vi "Tank.vi"() -> ()   [LabVIEW 2018]
panel:
  out "Remplissage":u16
  in  "Débit":u16(slide) scale=0.0..10.0
  in  "Consigne":u16(slide) max=1 step=1 scale=1.0..1000.0
  out "Tank":u16(slide) scale=0.0..1000.0
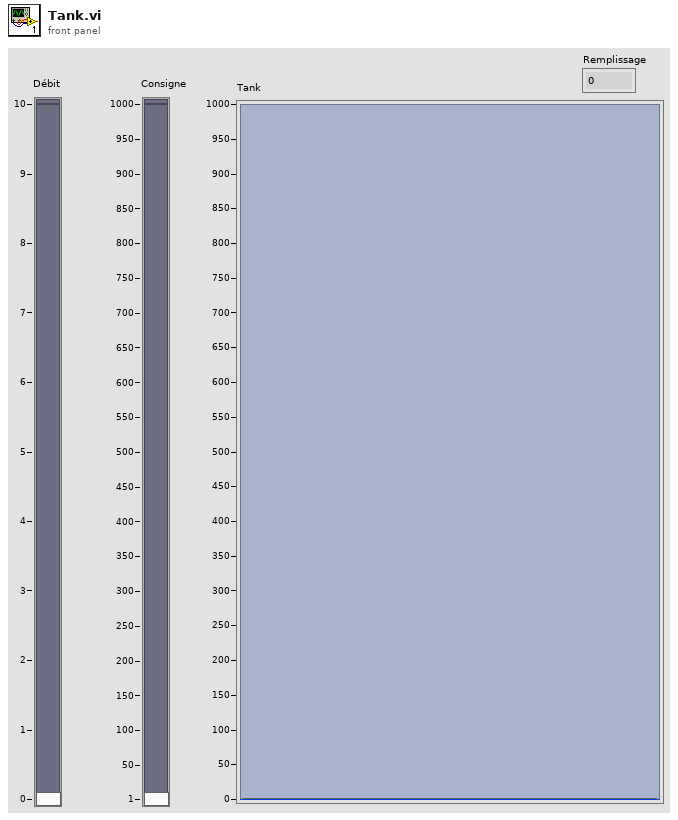
[diagram p1: front panel]
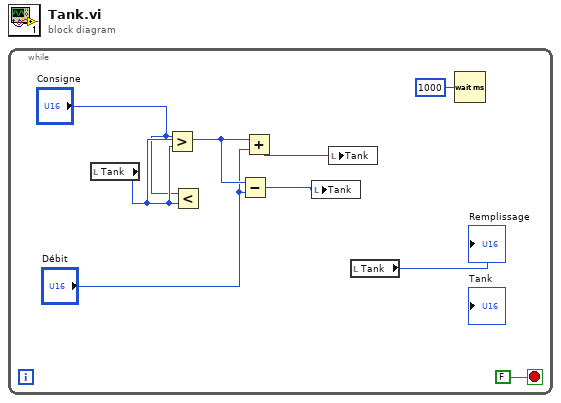
[diagram p0: block diagram]
diagram:
  n1 = while {
    stop <- FALSE stop-if-true
    n2 = local read "Tank"() -> (w6:u16)
    n3 = Greater?(x="Consigne", y=w6) -> ()  [unwired: 1 out]
    n4 = Less?(x="Consigne", y=w6) -> ()  [unwired: 1 out]
    n5 = Subtract(x=w6, y="Débit") -> (x-y=w8:u16)
    n6 = Add(x=w6, y="Débit") -> (x+y=w7:u16)
    n7 = local write "Tank"(w8) -> ()
    n8 = local write "Tank"(w7) -> ()
    n9 = local read "Tank"() -> (→"Remplissage":u16)
    n10 = Wait (ms)(milliseconds to wait=u32 1000) -> ()  [unwired: 1 out]
  }
